vi "HoloPy_test.vi"() -> ()   [LabVIEW 2023, in "holoTracker.lvlib"]
uses:
  holoTracker.lvlib
  subVis/HologramInfo.ctl
  CCL_parameters.ctl
panel:
  in  "ParametersIN":T3 {"Holo parameters"."Holo size X" format="%.0g"; "Holo parameters"."pixel size" format="%#_6e"; "Holo parameters"."wavelength" format="%#_6e"; "CCL parameters"."max voxel" min=0.0 max=0.0; "CCL parameters"."min voxel" min=1.0 max=100.0; "CCL parameters"."Threshold ( N x Standard deviation)" min=1.0 max=100.0}
  out "ParametersOUT":T3 {"Holo parameters"."Holo size X" format="%.0g"; "Holo parameters"."pixel size" format="%#_6e"; "Holo parameters"."wavelength" format="%#_6e"; "CCL parameters"."max voxel" min=0.0 max=0.0; "CCL parameters"."min voxel" min=1.0 max=100.0; "CCL parameters"."Threshold ( N x Standard deviation)" min=1.0 max=100.0}
  out "return value":string
  in  "error in (no error)":errorcluster
  in  "Python version":string="3.10"
  out "error out":errorcluster
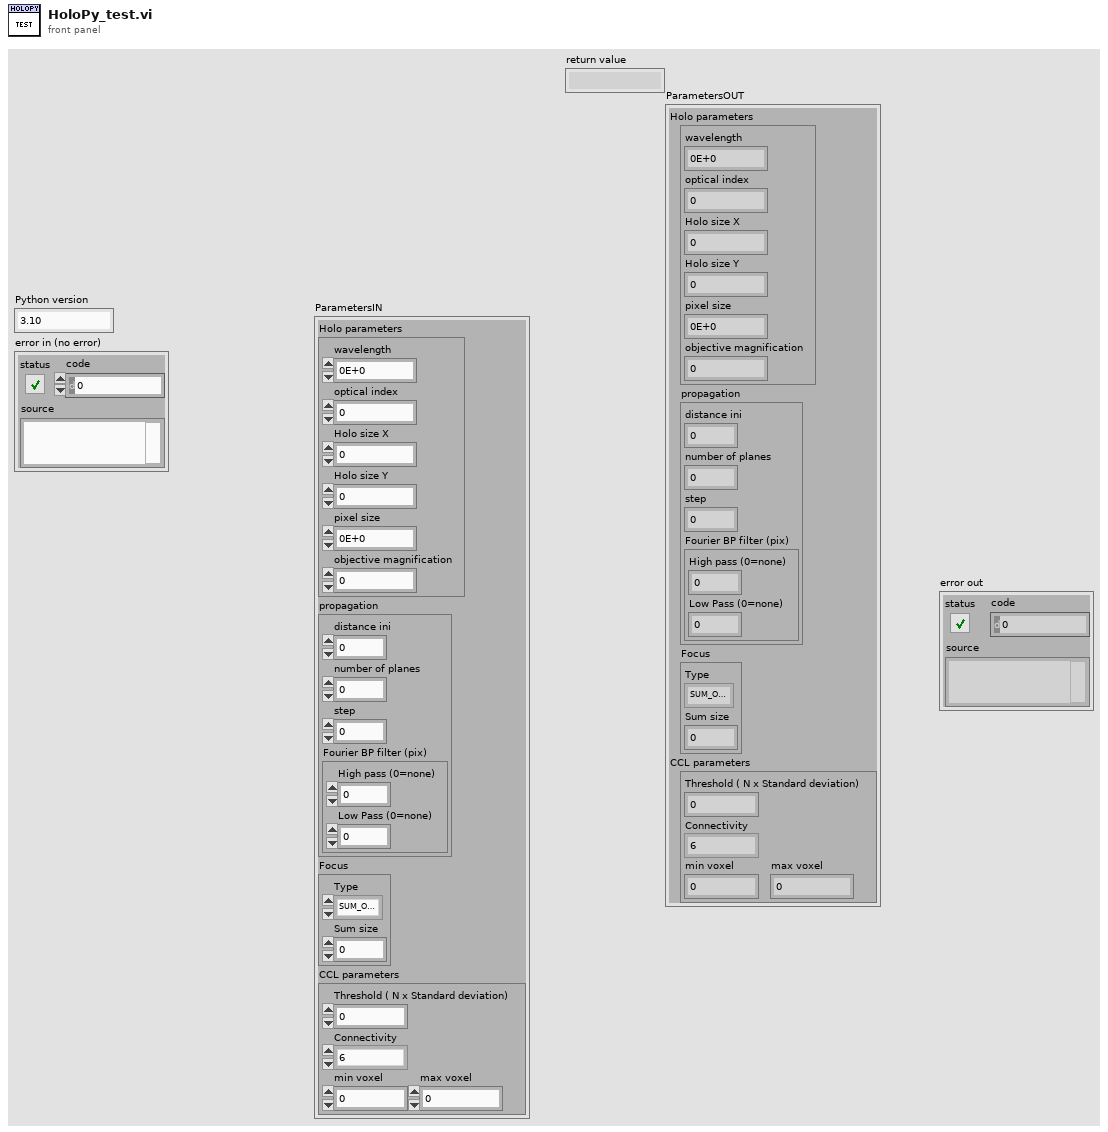
[diagram p1: front panel]
types:
  T1 = typedef "holoTracker.lvlib/HologramInfo.ctl" = cluster{"wavelength":sgl, "optical index":sgl, "Holo size X":i32, "Holo size Y":i32, "pixel size":sgl, "objective magnification":sgl}
  T2 = typedef "CCL_parameters.ctl" = cluster{"Threshold ( N x Standard deviation)":dbl, "Connectivity":enum16{"6", "18", "26"}, "min voxel":dbl, "max voxel":dbl}
  T3 = cluster{"Holo parameters":T1, "propagation":cluster{"distance ini":dbl, "number of planes":i32, "step":dbl, "Fourier BP filter (pix)":cluster{"High pass (0=none)":dbl, "Low Pass (0=none)":dbl}}, "Focus":cluster{"Type":enum16{"SUM_OF_INTENSITY", "SUM_OF_LAPLACIAN", "SUM_OF_VARIANCE", "TENENGRAD"}, "Sum size":i32}, "CCL parameters":T2}
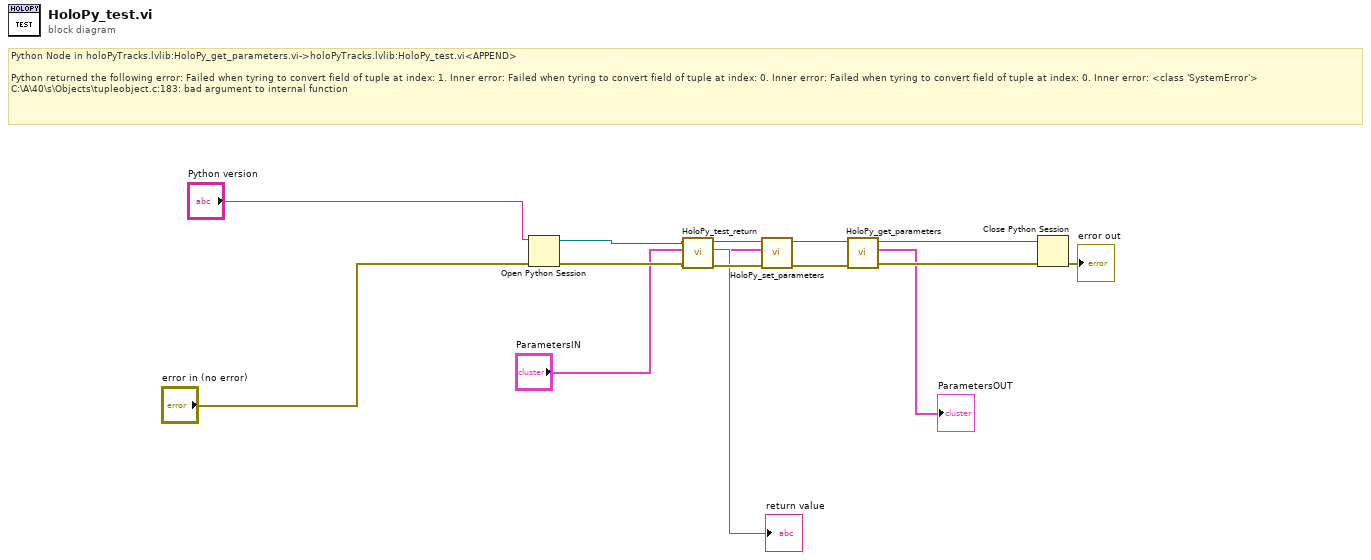
[diagram p0: block diagram]
diagram:
  # "Python Node in holoPyTracks.lvlib:HoloPy_get_parameters.vi->holoPyTracks.lvlib:HoloPy_test.vi<APPEND>\n\nPython returned the following error: Failed when tyring to convert field of tuple at index: 1. Inner error: Failed when tyring to convert field of tuple at index: 0. Inner error: Failed when tyring to convert field of tuple at index: 0. Inner error: <class 'SystemError'>\nC:\\A\\40\\s\\Objects\\tupleobject.c:183: bad argument to internal function"
  n1 = Open Python Session(python version="Python version", 3:"error in (no error)") -> (session out=w11:refnum<k35>, error out=w10:errorcluster)  [unwired: 1 in]
  n2 = call "HoloPy_test_return.vi"("error in (no error)"=w10, "Refnum in"=w11) -> ("error out"=w9:errorcluster, "return value"=→"return value":string, "Refnum out"=w8:refnum<k35>)  [unwired: 7 in]
  n3 = call "HoloPy_set_parameters.vi"("error in (no error)"=w9, "ParametersIN"="ParametersIN", "session in"=w8) -> ("error out"=w7:errorcluster, "Refnum out"=w6:refnum<k35>)  [unwired: 6 in, 1 out]
  n4 = call "HoloPy_get_parameters.vi"("error in (no error)"=w7, "session in"=w6) -> ("error out"=w4:errorcluster, "ParametersOUT"=→"ParametersOUT":T3, "Refnum out"=w5:refnum<k35>)  [unwired: 7 in]
  n5 = Close Python Session(session in=w5, error in=w4) -> (11:→"error out":errorcluster)
